vi "Convert_No._to_String_ADAM.vi"(1 "Input number":dbl format="%.12f", 2 "Ch Description":T1={"Ch Name"="", "Type"="", "Function"=enum."Analogue Input", "Ch State"=enum."On", "Calibration type"=enum."Raw", "A"=0.0, "B"=0.0, "C"=0.0, "D"=0.0, "Comments"="", "Address"={"Main"=0, "Ch."=0, "Sub"=0, "Port Name"=""}, "String"="", "Duty"=65535} {"Duty" format="%.0b"; "D" format="%#_5g"; "C" format="%#_5g"; "B" format="%#_5g"; "A" format="%#_5g"}) -> (0 "Output sting":string)   [LabVIEW 2012]
uses:
  ADAM Controls/Ch_description_ADAM.ctl
  ADAM Controls/Module_type_ADAM.ctl
  ADAM Controls/Function_ADAM.ctl
  ADAM Controls/Channel_State.ctl
  ADAM Controls/Calib_type_ADAM.ctl
  ADAM Controls/Address.ctl
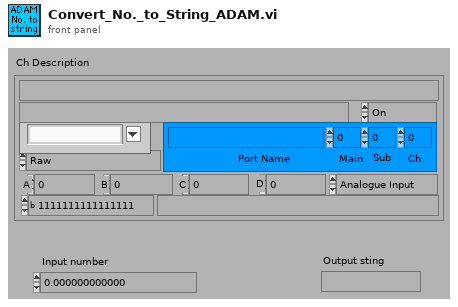
[diagram p1: front panel]
types:
  T1 = typedef "Ch_description_ADAM.ctl" = cluster{"Ch Name":string, "Type":T2, "Function":T3, "Ch State":T4, "Calibration type":T5, "A":dbl, "B":dbl, "C":dbl, "D":dbl, "Comments":string, "Address":T6, "String":string, "Duty":u16}
  T2 = typedef "Module_type_ADAM.ctl" = string
  T3 = typedef "Function_ADAM.ctl" = enum16{"Analogue Input", "Digital Input", "Event counter", "Event rate", "Analogue Output", "Digital Output", "Relay Output"}
  T4 = typedef "Channel_State.ctl" = enum16{"On", "Off", "Always On", "Always Off"}
  T5 = typedef "Calib_type_ADAM.ctl" = enum16{"Raw", "Bx + A", "Cx^2 + Bx + A", "Dx^3 + Cx^2 + Bx + A", "In Band", "Hi-Tec Q", "Hi-Tec M_dot", "Text"}
  T6 = typedef "Address.ctl" = cluster{"Main":i32, "Ch.":i32, "Sub":i32, "Port Name":string}
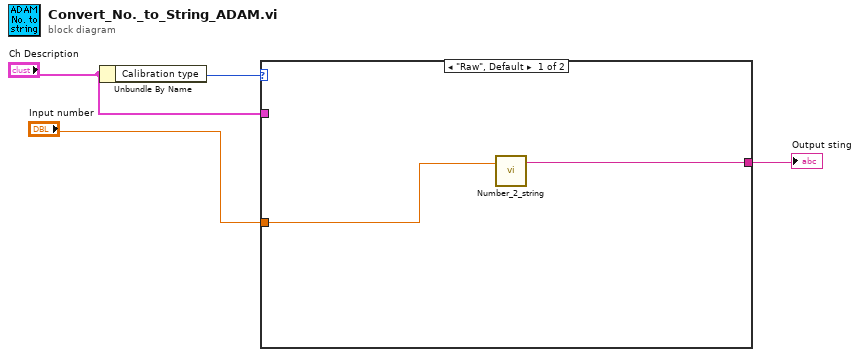
[diagram p0: block diagram]
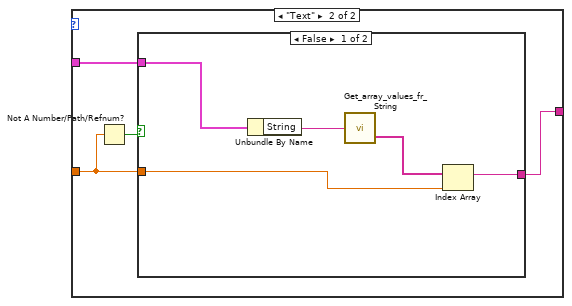
[diagram p2: hidden frame]
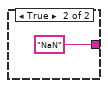
[diagram p3: hidden frame]
diagram:
  n1 = Unbundle By Name("Ch Description") -> ("Calibration type"=w2:T5)
  n2 = case shown="\"Raw\", Default" w2 {
    tunnel: "Input number" -> [w6 w9]
    tunnel: [w5 w10] -> w4
    tunnel: "Ch Description" -> [_ w7]
    frame "Raw", Default {
      n3 = call "Number_2_string.vi"("number"=w6) -> ("String"=w5:string)  [unwired: 1 in]
    }
    frame "Text" {
      n4 = Not A Number/Path/Refnum?(number/path/refnum=w9) -> (NaN/Path/Refnum?=w8:bool)
      n5 = case shown="False" w8 {
        tunnel: [w13 "NaN" ("Output")] -> w10
        tunnel: w9 -> [w14 _]
        tunnel: w7 -> [w11 _]
        frame False {
          n6 = Unbundle By Name(w11) -> ("String"=w12:string)
          n7 = call "Get_array_values_fr_String.vi"("String Value"=w12) -> ("String array"=w15:string[])  [unwired: 1 out]
          n8 = Index Array(array=w15, index=w14) -> (element=w13:string)
        }
        frame True {
        }
      }
    }
  }
  "Output sting" <- w4
